vi "Untitled 10.vi"() -> ()   [LabVIEW 2014, in "AMS TS3472 Light Sensor.lvlib"]
uses:
  AMS TS3472 Light Sensor.lvlib
  AMS TCS3472.lvclass
panel:
  out "Address":u16=41 format="0x %.0x"
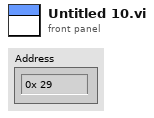
[diagram p1: front panel]
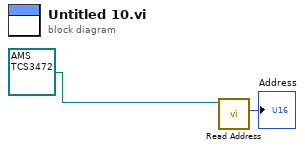
[diagram p0: block diagram]
diagram:
  n1 = call-dynamic "Read Address .vi"("AMS TS3472 in"=refnum<class "AMS TCS3472.lvclass"> refnum ("AMS TS3472 Light Sensor.lvlib:AMS TS3472.lvclass")) -> ("Address"=→"Address":u16)  [unwired: 8 in, 2 out]
